vi "Test_sqlite3QueryVIMScalarDoubleWorks_NoError.vi"(8 "error in (no error)":errorcluster, 11 "TestCase in":refnum<class "Test sqlite3.lvclass">) -> (0 "error out":errorcluster, 3 "TestCase out":refnum<class "Test sqlite3.lvclass">)   [LabVIEW 2020, in "Test sqlite3.lvclass"]
uses:
  Test sqlite3.lvclass
  Test sqlite3.lvclass/Test sqlite3.ctl
  <vilib>/addons/_JKI Toolkits/VI Tester/TestCase.llb/TestCase.lvclass
  45a547b6-e4c0-49d6-ab78-a1d3563bf804.vi
  externals/sqlite3/Source/sqlite3.lvclass
  externals/database-interface/IDatabase/IDatabase/IDatabase.lvclass
  C:/Program Files/National Instruments/LabVIEW 2020/vi.lib/addons/_JKI Toolkits/VI Tester/TestCase.llb/TestCase.lvclass
  C:/Users/Fred.Guo/Desktop/Database-configuration/externals/database-interface/Test/Test sqlite3/Test sqlite3.lvclass
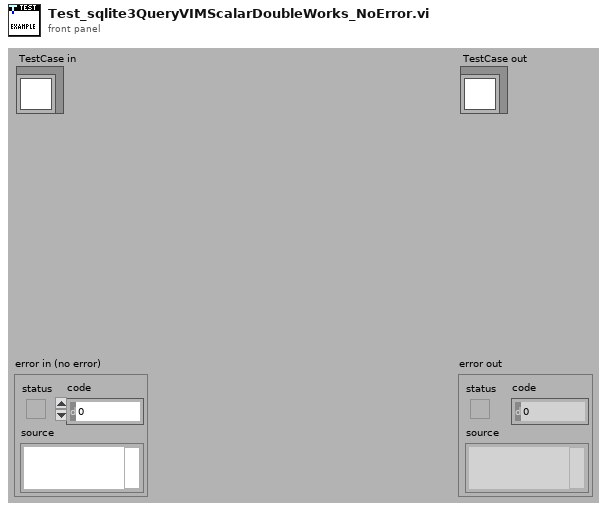
[diagram p1: front panel]
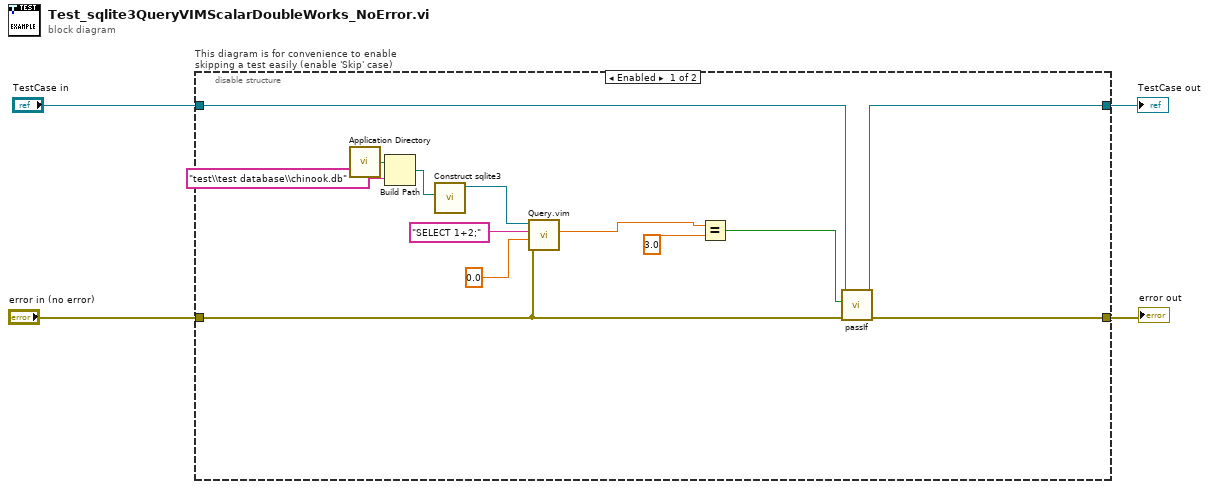
[diagram p0: block diagram]
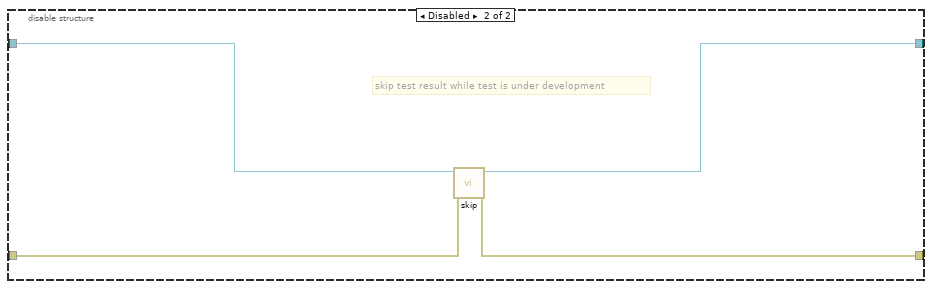
[diagram p2: hidden frame]
diagram:
  n1 = disable-structure "This diagram is for convenience to enable skipping a test easily (enable 'Skip' case)" shown="Enabled" {
    disable-tunnel: "TestCase in" -> [w15 w21]
    disable-tunnel: [w17 w19] -> w1
    disable-tunnel: [w16 w20] -> w3
    disable-tunnel: "error in (no error)" -> [w14 w18]
    frame Enabled {
      n2 = call <vilib>:"Application Directory.vi"() -> ("Application Directory"=w11:path)
      n3 = Build Path(base path=w11, name or relative path="test\\test database\\chinook.db") -> (appended path=w12:path)
      n4 = call "Construct sqlite3.vi"("DatabaseFilePath"=w12) -> ("sqlite3 out"=w7:refnum<class "sqlite3.lvclass">)  [unwired: 9 in, 1 out]
      n5 = call "Query.vim"("error in (no error)"=w14, "Type and Default"=0.0 ("y"), "Query string"="SELECT 1+2;", "IDatabase in"=w7) -> ("Result"=w6:dbl)  [unwired: 5 in, 2 out]
      n6 = Equal?(x=w6, y=3.0) -> (x = y?=w13:bool)
      n7 = call-dynamic "passIf.vi"("error in (no error)"=w14, "pass"=w13, "TestCase in"=w15) -> ("error out"=w16:errorcluster, "TestCase out"=w17:refnum<class "Test sqlite3.lvclass">)  [unwired: 7 in]
    }
    frame Disabled {
      # "skip test result while test is under development"
      n8 = call <vilib>:"skip.vi"("error in (no error)"=w18, "TestCase in"=w21) -> ("error out"=w20:errorcluster, "TestCase out"=w19:refnum<class "Test sqlite3.lvclass">)  [unwired: 8 in]
    }
  }
  "error out" <- w3
  "TestCase out" <- w1
